vi "sim.vi"() -> ()   [LabVIEW 2019]
uses:
  <vilib>/ptbypt/NI_PtbyPt.lvlib
panel:
  out "Waveform Graph":dbl[](graph)
  out "Waveform Chart 4":dbl(graph)
  in  "stop after":i32
  in  "milliseconds to wait":u32=50
  in  "stop":bool
  out "Boolean":bool
  in  "Periods Off":i32
  in  "Periods on":i32
  in  "Q Value":dbl
  in  "energy in per cycle":dbl
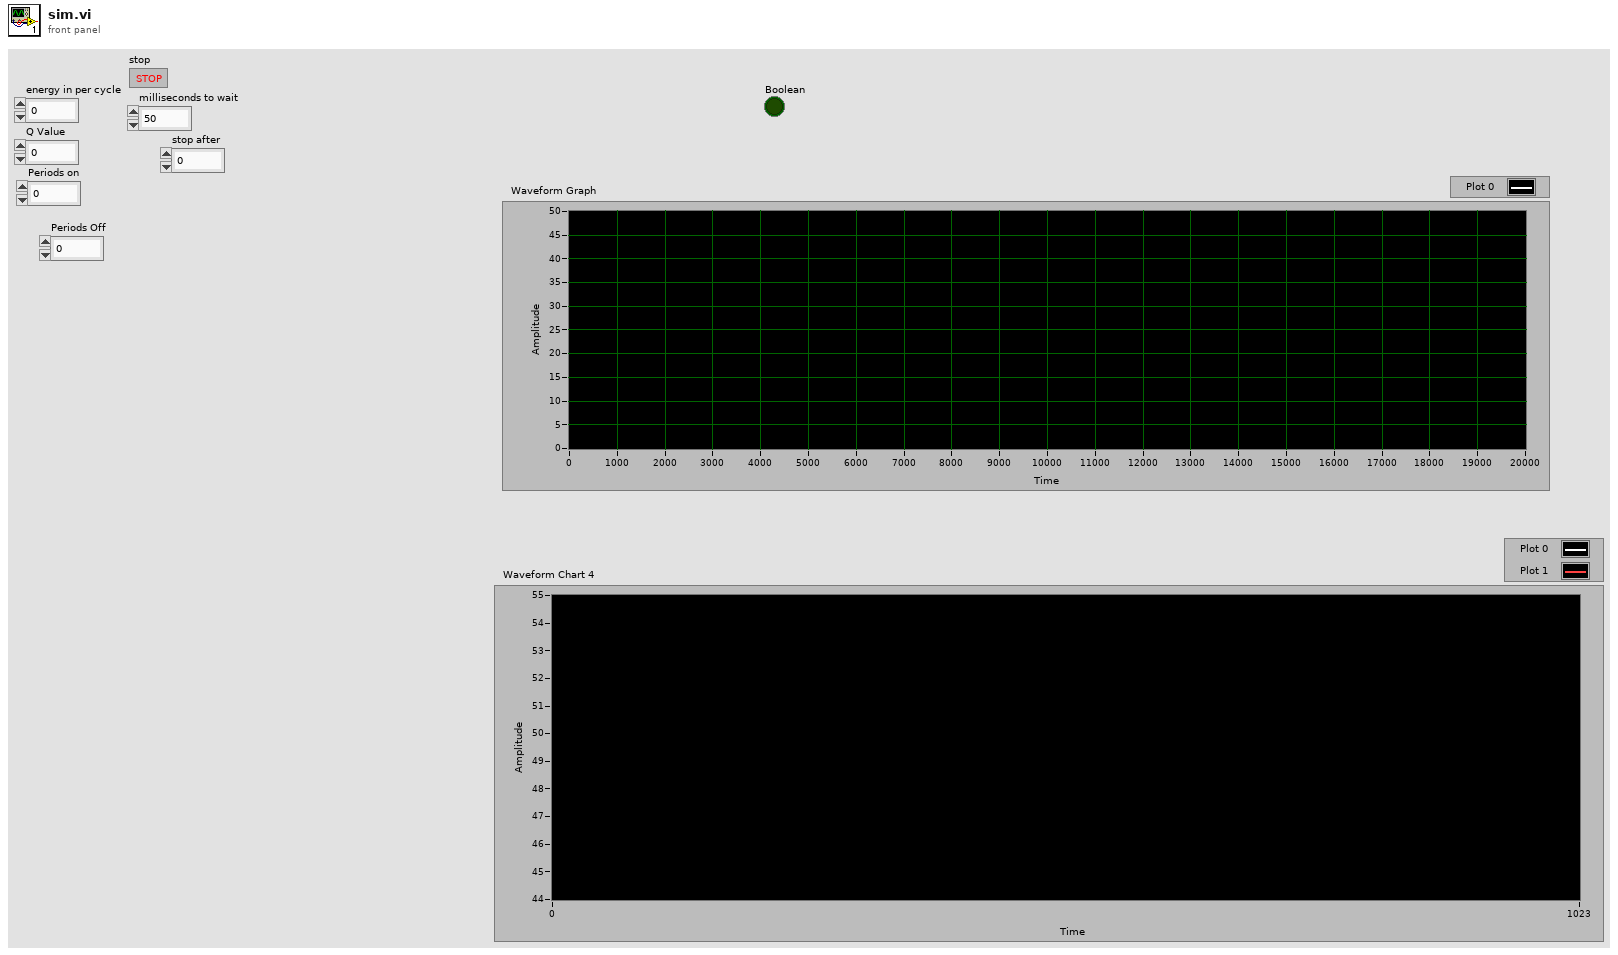
[diagram p1: front panel]
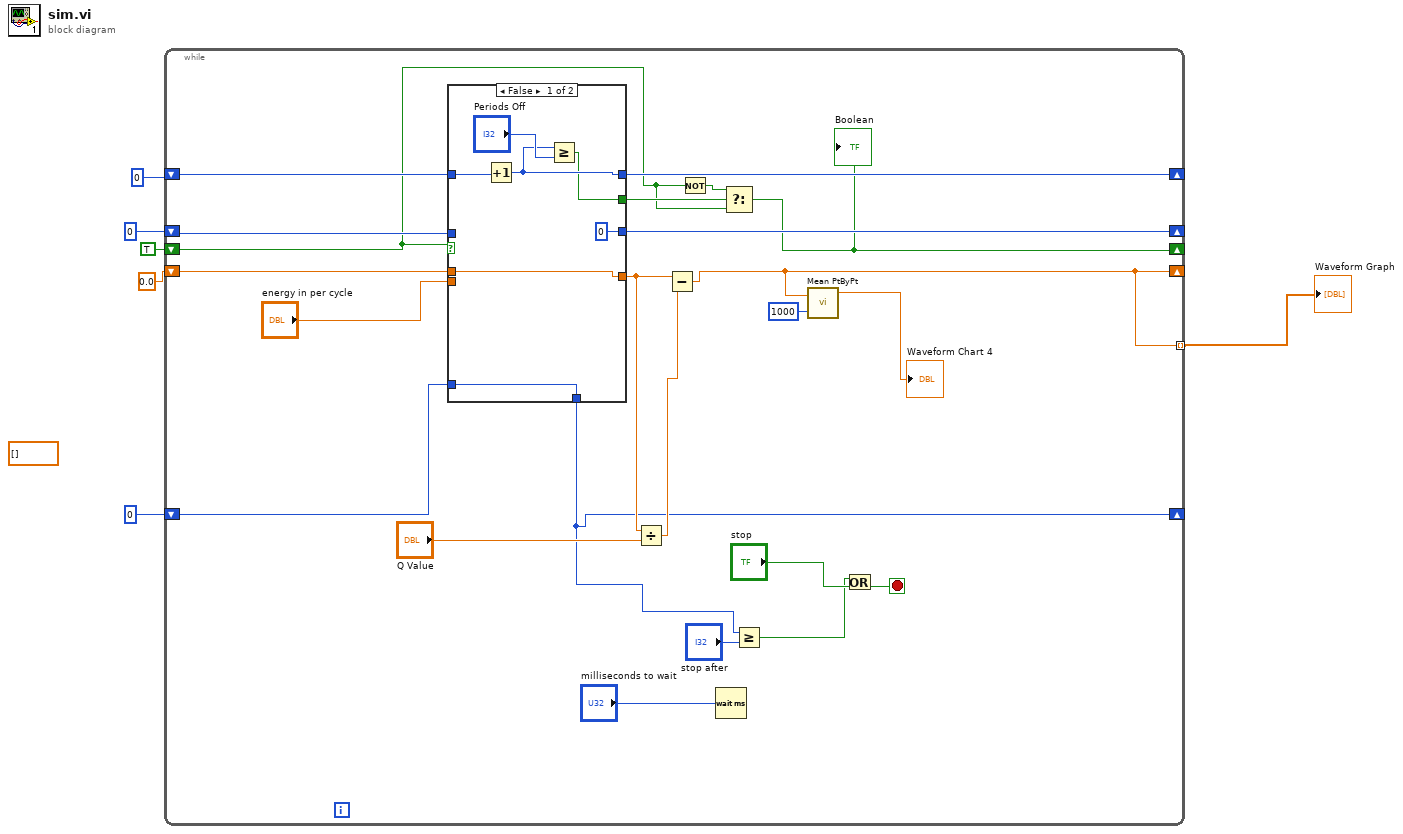
[diagram p0: block diagram]
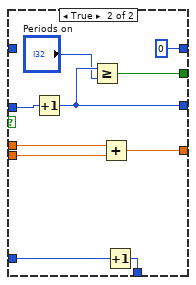
[diagram p2: hidden frame]
diagram:
  (unwired) dbl[] [] ("History Data")
  n1 = while {
    shift-right: [w7] -> _
    shift-left: 0.0 -> [w28]
    shift-right: [w24] -> _
    shift-left: 0 -> [w23]
    shift-right: [w17] -> _
    shift-left: TRUE -> [w18]
    shift-right: [w21] -> _
    shift-left: 0 -> [w22]
    shift-right: [w10] -> _
    shift-left: 0 -> [w14]
    tunnel: [w7] -> w1 mode=indexing
    stop <- w12 stop-if-true
    n2 = case shown="False" w18 {
      tunnel: "energy in per cycle" -> [_ w46]
      tunnel: w28 -> [w36 w37]
      tunnel: [w36 w45] -> w25
      tunnel: w23 -> [_ w44]
      tunnel: [0 w43] -> w24
      tunnel: w22 -> [w34 _]
      tunnel: [w32 0] -> w21
      tunnel: [w31 w40] -> w19
      tunnel: w14 -> [w30 w39]
      tunnel: [w30 w38] -> w10
      frame False {
        n3 = Increment(x=w34) -> (x+1=w32:i32)
        n4 = Greater Or Equal?(x=w32, y="Periods Off") -> (x >= y?=w31:bool)
      }
      frame True {
        n5 = Increment(x=w44) -> (x+1=w43:i32)
        n6 = Greater Or Equal?(x=w43, y="Periods on") -> (x >= y?=w40:bool)
        n7 = Add(x=w37, y=w46) -> (x+y=w45:dbl)
        n8 = Increment(x=w39) -> (x+1=w38:i32)
      }
    }
    n9 = Divide(x=w25, y="Q Value") -> (x/y=w26:dbl)
    n10 = Subtract(x=w25, y=w26) -> (x-y=w7:dbl)
    n11 = Not(x=w18) -> (.not. x?=w20:bool)
    n12 = Wait (ms)(milliseconds to wait="milliseconds to wait") -> ()  [unwired: 1 out]
    n13 = Select(t=w20, s=w19, f=w18) -> (s? t:f=w17:bool)
    "Boolean" <- w17
    n14 = Greater Or Equal?(x=w10, y="stop after") -> (x >= y?=w11:bool)
    n15 = call <vilib>:"Mean PtByPt.vi"("x"=w7, "sample length"=1000) -> ("mean"=→"Waveform Chart 4":dbl)  [unwired: 2 in, 1 out]
    n16 = Or(x=w11, y="stop") -> (x .or. y?=w12:bool)
  }
  "Waveform Graph" <- w1
